vi "Add_to_sequence_SubVI_v1.vi"(1 "Delay [us]":dbl, 2 "Pulse length [us]":dbl, 3 "Channel number":i32, 4 "Array sequence in":cluster{"Timing 0":dbl[]}[](array[cluster])) -> (0 "Array sequence out":cluster{"Timing 0":dbl[]}[](array[cluster]))   [LabVIEW 2021]
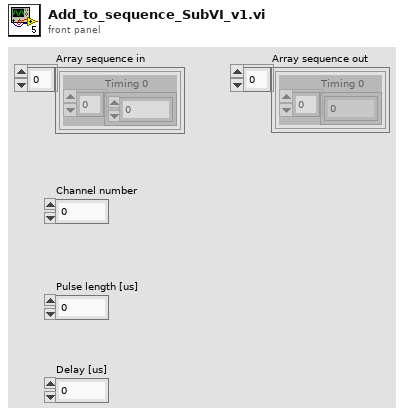
[diagram p1: front panel]
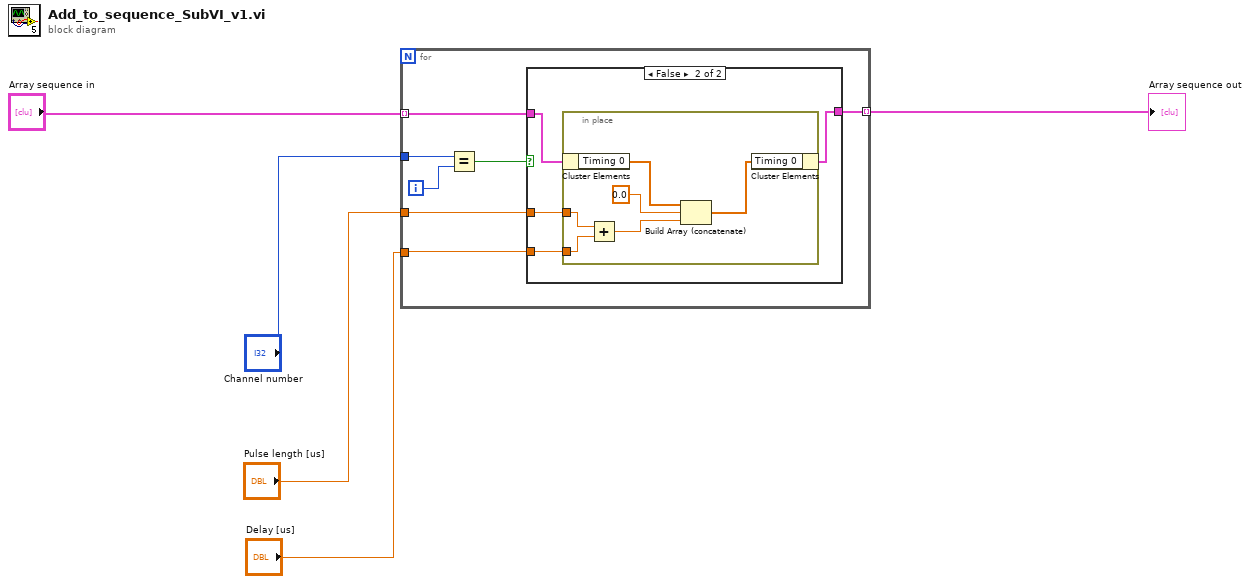
[diagram p0: block diagram]
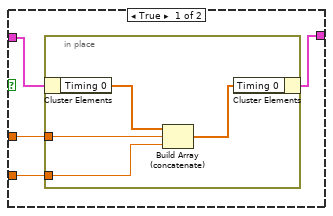
[diagram p2: hidden frame]
diagram:
  n1 = for {
    tunnel: "Array sequence in" -> [w9] mode=indexing
    tunnel: "Channel number" -> [w12]
    tunnel: "Pulse length [us]" -> [w8]
    tunnel: [w7] -> w5 mode=indexing
    tunnel: "Delay [us]" -> [w6]
    i -> [w11]
    n2 = Equal?(x=w12, y=w11) -> (x = y?=w10:bool)
    n3 = case shown="False" w10 {
      tunnel: w9 -> [w16 w24]
      tunnel: w8 -> [w15 w23]
      tunnel: [w14 w22] -> w7
      tunnel: w6 -> [w13 w21]
      frame True {
        n4 = in-place {
          in-place-border: w15 -> [w20]
          in-place-border: w13 -> [w17]
          n5 = in-place-cluster #1(w16) -> ("Timing 0"=w19:dbl[])
          n6 = Build Array (concatenate)(w19, w20, w17) -> (w18:dbl[])
          n7 = in-place-cluster #1("Timing 0"=w18) -> (w14:cluster{"Timing 0":dbl[]})
        }
      }
      frame False {
        n8 = in-place {
          in-place-border: w23 -> [w27]
          in-place-border: w21 -> [w26]
          n9 = in-place-cluster #2(w24) -> ("Timing 0"=w30:dbl[])
          n10 = Add(x=w27, y=w26) -> (x+y=w25:dbl)
          n11 = Build Array (concatenate)(w30, 0.0 ("element"), w25) -> (w29:dbl[])
          n12 = in-place-cluster #2("Timing 0"=w29) -> (w22:cluster{"Timing 0":dbl[]})
        }
      }
    }
  }
  "Array sequence out" <- w5
